vi "Exemple_Metrics_Pairwise_Nan_Euclidean_Distances.vi"() -> ()   [LabVIEW 2020]
uses:
  Objet/6 - Datasets Transformation/6.8 - Pairwise metrics, Affinities and Kernels/Nan_euclidean_distances/Nan_euclidean_distances.vi
panel:
  in  "nan_euclidean_distances":T1={"squared"=FALSE, "missing_values"="nan", "copy"=TRUE}
  in  "error in":errorcluster caption="entrée d'erreur"
  in  "Y":string[][](array[string])=[["1", "2"], ["0", "3"]]
  in  "X":string[][](array[string])=[["0", "1"], ["1", "nan"]]
  out "Data":T2
  out "error out":errorcluster caption="sortie d'erreur"
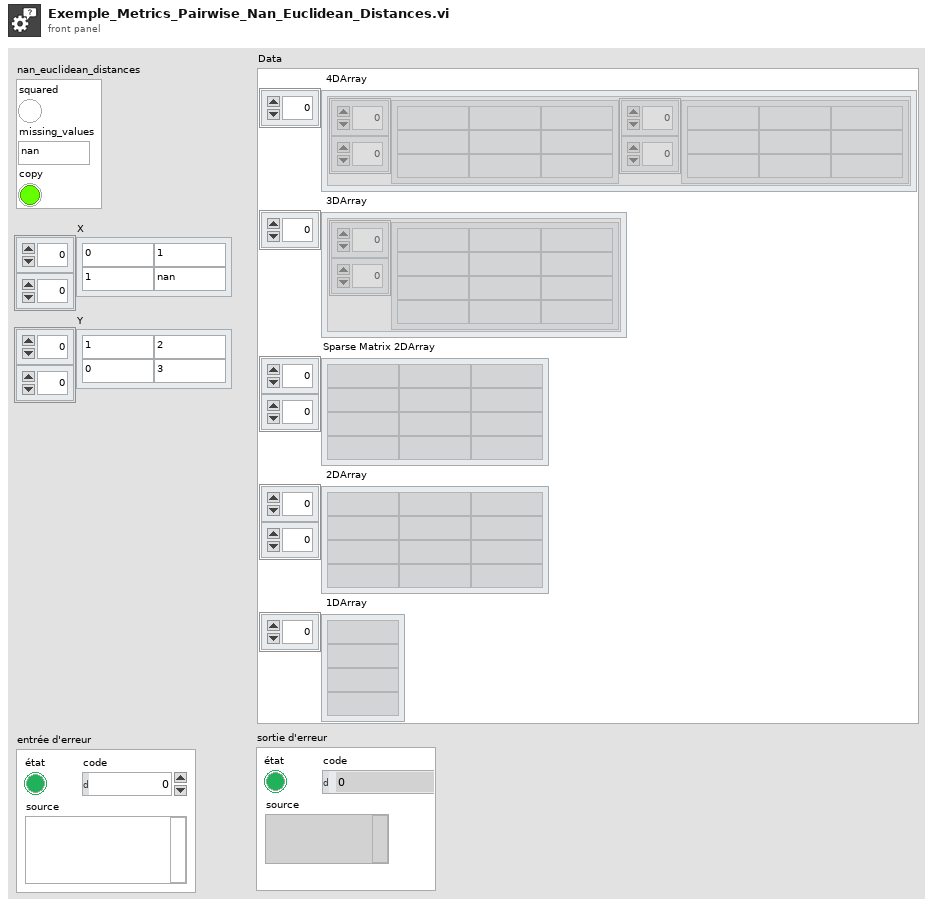
[diagram p1: front panel]
types:
  T1 = cluster{"squared":bool, "missing_values":string, "copy":bool}
  T2 = cluster{" 4DArray":cluster{"1":string[][], "2":string[][]}[], " 3DArray":cluster{"Tableau":string[][]}[], "Sparse Matrix 2DArray":string[][], " 2DArray":string[][], " 1DArray":string[]}
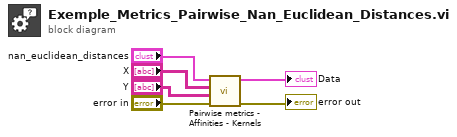
[diagram p0: block diagram]
diagram:
  n1 = call-poly "Pairwise metrics - Affinities - Kernels.vi"("error in"="error in", "Y"="Y", "X"="X", "nan_euclidean_distances"="nan_euclidean_distances") -> ("error out"=→"error out":errorcluster, "Data"=→"Data":T2)  [unwired: 6 in]
